vi "Is External Source.vi"(11 "BluelinesRedlines Source in":refnum<class "BluelinesRedlines Source.lvclass">) -> (2 "External Source":bool)   [LabVIEW 2020, in "VolatusGUI.lvlib" / "BluelinesRedlines Source.lvclass"]
uses:
  BluelinesRedlines Source.lvclass
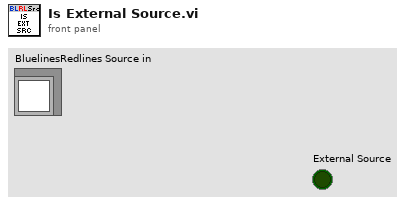
[diagram p1: front panel]
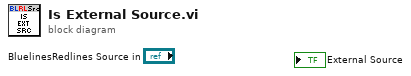
[diagram p0: block diagram]
diagram:
